vi "Static Lock.vi"(9 "Page to Lock [03-0F]":i32 format="%x", 11 "PN532 COM Port":refnum<visa-resource-name>) -> (0 "Error out":errorcluster, 2 "Succeeded":bool, 3 "PN532 COM Port Out":refnum<visa-resource-name>)   [LabVIEW 2012, in "NFC Driver.lvlib"]
uses:
  NFC Driver.lvlib
panel:
  out "result string":string
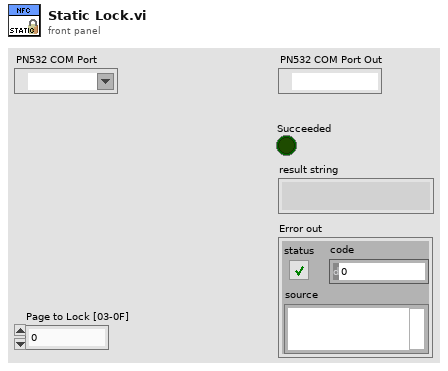
[diagram p1: front panel]
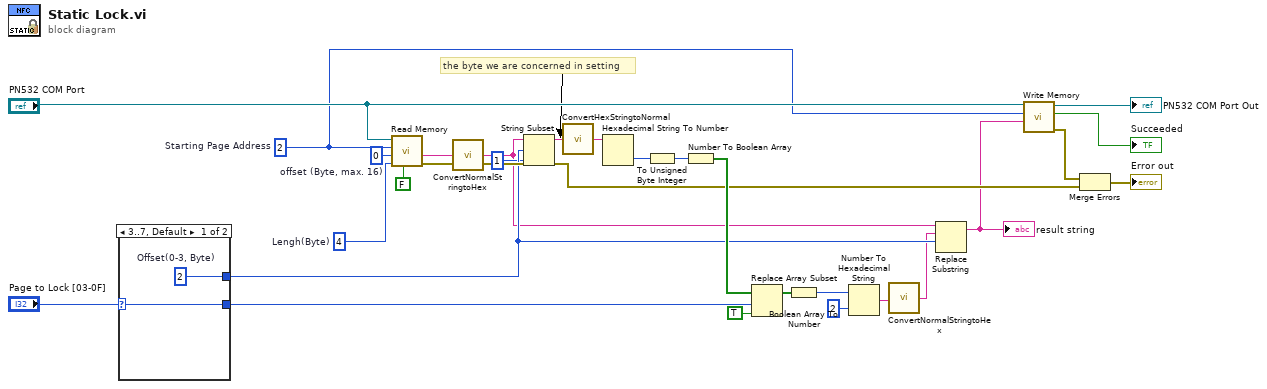
[diagram p0: block diagram]
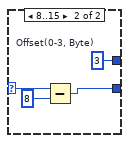
[diagram p2: hidden frame]
diagram:
  w11 = 0  # offset (Byte, max. 16)
  w24 = 4  # Lengh(Byte)
  w4 = 2  # Starting Page Address
  # "the byte we are concerned in setting"
  n1 = case shown="3..7, Default" "Page to Lock [03-0F]" {
    selector: "Page to Lock [03-0F]" -> [w29 w33]
    tunnel: [w30 w34] -> w10
    tunnel: [w29 w32] -> w16
    frame 3..7, Default {
      w30 = 2  # Offset(0-3, Byte)
    }
    frame 8..15 {
      w34 = 3  # Offset(0-3, Byte)
      n2 = Subtract(x=w33, y=8) -> (x-y=w32:i32)
    }
  }
  n3 = call "Read Memory.vi"("Reverse Output[F]"=FALSE, "length (Byte, max. 16)"=w24, "offset (Byte, max. 16)"=w11, "Page Address"=w4, "PN532 COM Port"="PN532 COM Port") -> ("error out"=w18:errorcluster, "Selected substring (HEX)"=w3:string)  [unwired: 2 in, 3 out]
  n4 = call "ConvertNormalStringtoHex.vi"("Normal String"=w3) -> ("Hex String"=w7:string)
  n5 = String Subset(string=w7, offset (0)=w10, length (rest)=1 ("length (rest)")) -> (substring=w13:string)
  n6 = call "ConvertHexStringtoNormal.vi"("Hex String"=w13) -> ("Normal String"=w6:string)
  n7 = Hexadecimal String To Number(string=w6) -> (number=w23:u32)  [unwired: 2 in, 1 out]
  n8 = To Unsigned Byte Integer(number=w23) -> (unsigned 8bit integer=w14:u8)
  n9 = Number To Boolean Array(number=w14) -> (Boolean array=w22:bool[])
  n10 = Replace Array Subset(array=w22, new element=TRUE ("new element/subarray"), index=w16) -> (w17:bool[])
  n11 = Boolean Array To Number(Boolean array=w17) -> (number=w21:u32)
  n12 = Number To Hexadecimal String(1:i16 2 ("width (-)"), 2:w21) -> (0:w9:string)
  n13 = call "ConvertNormalStringtoHex.vi"("Normal String"=w9) -> ("Hex String"=w5:string)
  n14 = Replace Substring(3:w10, 4:w5, 5:w7) -> (1:w12:string)  [unwired: 1 in, 1 out]
  "result string" <- w12
  n15 = call "Write Memory.vi"("Data to write (HEX, max 16 bytes)"=w12, "Page Address"=w4, "PN532 COM Port"="PN532 COM Port") -> ("Error Out"=w19:errorcluster, "Succesful?"=→"Succeeded":bool, "PN532 COM Port Out"=→"PN532 COM Port Out":refnum<visa-resource-name>)  [unwired: 6 in]
  n16 = Merge Errors(w19, w18) -> (→"Error out":errorcluster)
